vi "Identify VI Path.vi"(7 "ID":string, 11 "State Data":T1) -> (3 "VI Path":path)   [LabVIEW 2018]
doc: "Identifies whether to take the Assert VI path or the Temp VI path for adding to the calling vi"
uses:
  Insert Process Data.ctl
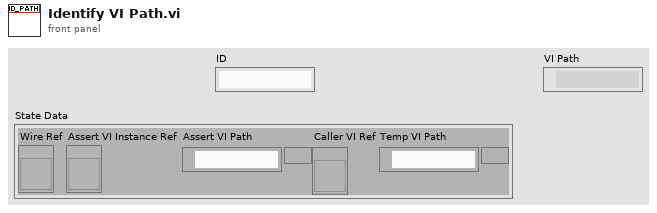
[diagram p1: front panel]
types:
  T1 = typedef "Insert Process Data.ctl" = cluster{"Wire Ref":refnum<vi>, "Assert VI Instance Ref":refnum<vi>, "Assert VI Path":path, "Caller VI Ref":refnum<vi>, "Temp VI Path":path}
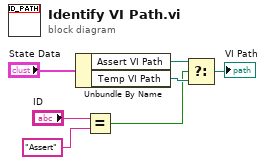
[diagram p0: block diagram]
diagram:
  n1 = Unbundle By Name("State Data") -> ("Assert VI Path"=w5:path, "Temp VI Path"=w6:path)
  n2 = Equal?(x="ID", y="Assert" ("regular expression")) -> (x = y?=w3:bool)
  n3 = Select(t=w5, s=w3, f=w6) -> (s? t:f=→"VI Path":path)
